vi "FFT_CALCULATOR.vi"(8 "Frame rate":i32, 9 "FFT size":i32, 11 "lm":dbl[](array[numeric])) -> (1 "Magnitude":dbl[](array[numeric]), 3 "lm-m":dbl[](array[numeric]), 4 "df":dbl format="%.2f", 6 "dt":dbl format="%.2f")   [LabVIEW 2015]
uses:
  <vilib>/Analysis/baseanly.llb/Mean (DBL).vi
  <vilib>/Analysis/2dsp.llb/Real FFT.vi
  <vilib>/Analysis/NI_AALPro.lvlib
  <vilib>/Analysis/NI_AALBase.lvlib
panel:
  out "Frequency Graph":dbl[](graph)
  out "Time Graph":dbl[](graph)
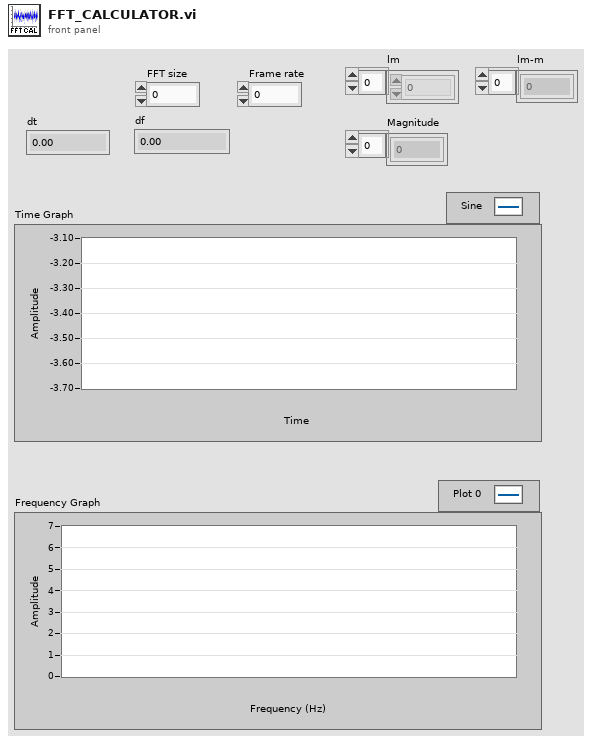
[diagram p1: front panel]
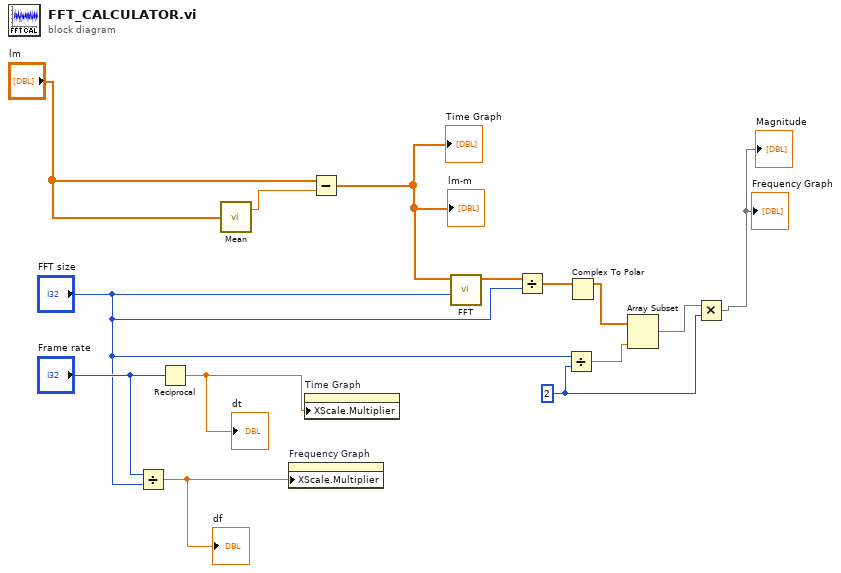
[diagram p0: block diagram]
diagram:
  w9 = 2
  n1 = Divide(x="Frame rate", y="FFT size") -> (x/y=w6:dbl)
  "df" <- w6
  n2 = Reciprocal(x="Frame rate") -> (1/x=w8:dbl)
  "dt" <- w8
  n3 = call-poly <vilib>:"Mean.vi"("X"="lm") -> ("mean"=w1:dbl)  [unwired: 1 out]
  n4 = property on="Frequency Graph" class="WFGraph (strict)"("XScale.Multiplier"=w6) -> ()  [unwired: 2 in, 2 out]
  n5 = property on="Time Graph" class="WFGraph (strict)"("XScale.Multiplier"=w8) -> ()  [unwired: 2 in, 2 out]
  n6 = Subtract(x="lm", y=w1) -> (x-y=w2:dbl[])
  "Time Graph" <- w2
  "lm-m" <- w2
  n7 = call-poly <vilib>:"FFT.vi"("FFT size"="FFT size", "X"=w2) -> ("FFT {X}"=w14:cdb[])  [unwired: 8 in, 1 out]
  n8 = Divide(x=w14, y="FFT size") -> (x/y=w13:cdb[])
  n9 = Divide(x="FFT size", y=w9) -> (x/y=w10:dbl)
  n10 = Complex To Polar(r * e^(i*theta)=w13) -> (r=w12:dbl[])  [unwired: 1 out]
  n11 = Array Subset "Array Subset"(array=w12, length=w10) -> (w11:dbl[])  [unwired: 1 in]
  n12 = Multiply(x=w11, y=w9) -> (x*y=→"Frequency Graph" →"Magnitude":dbl[])
